vi "List Packages in SystemLink Feed.vi"(0 "SystemLink repo in":T1, 5 "feed name in":string, 11 "error in (no error)":errorcluster) -> (4 "SystemLink repo out":T1, 6 "feed name out":string, 8 "packages":string[][](table), 15 "error out":errorcluster)   [LabVIEW 2017, in "SystemLink_Repo_API.lvlib"]
doc: "Lists the packages for the specified feed.\n\nOutputs:\nPackages - This is a table (2D string array) that lists the packages in the specified feed. The table includes the name, version, filename, and package ID for each package."
uses:
  SystemLink_Repo_API.lvlib
  _support/systemlink repo.ctl
  <vilib>/httpClient/ClientHandle.ctl
  0c27402d-d134-44f2-9e9f-9c548188b8ee.vi
  73f63470-54eb-45b7-8baf-304f99d209d6.vi
  <vilib>/JDP Science/JSONtext/Find Multiple Items.vi
  <vilib>/JDP Science/JSONtext/String Subset.vi
  <vilib>/JDP Science/JSONtext/support/Strip Quotes and Unescape.vi
  <vilib>/JDP Science/JSONtext/Parsing/Parse Full Path or Item Name.vi
  <vilib>/JDP Science/JSONtext/Offset/Find Item Locations by Path.vi
  <vilib>/JDP Science/JSONtext/support/Unescape JSON string.vi
  <vilib>/JDP Science/JSONtext/JSON text to Variant.vi
  <vilib>/httpClient/LabVIEWHTTPClient.lvlib
panel:
  out "body":string
  out "headers":string
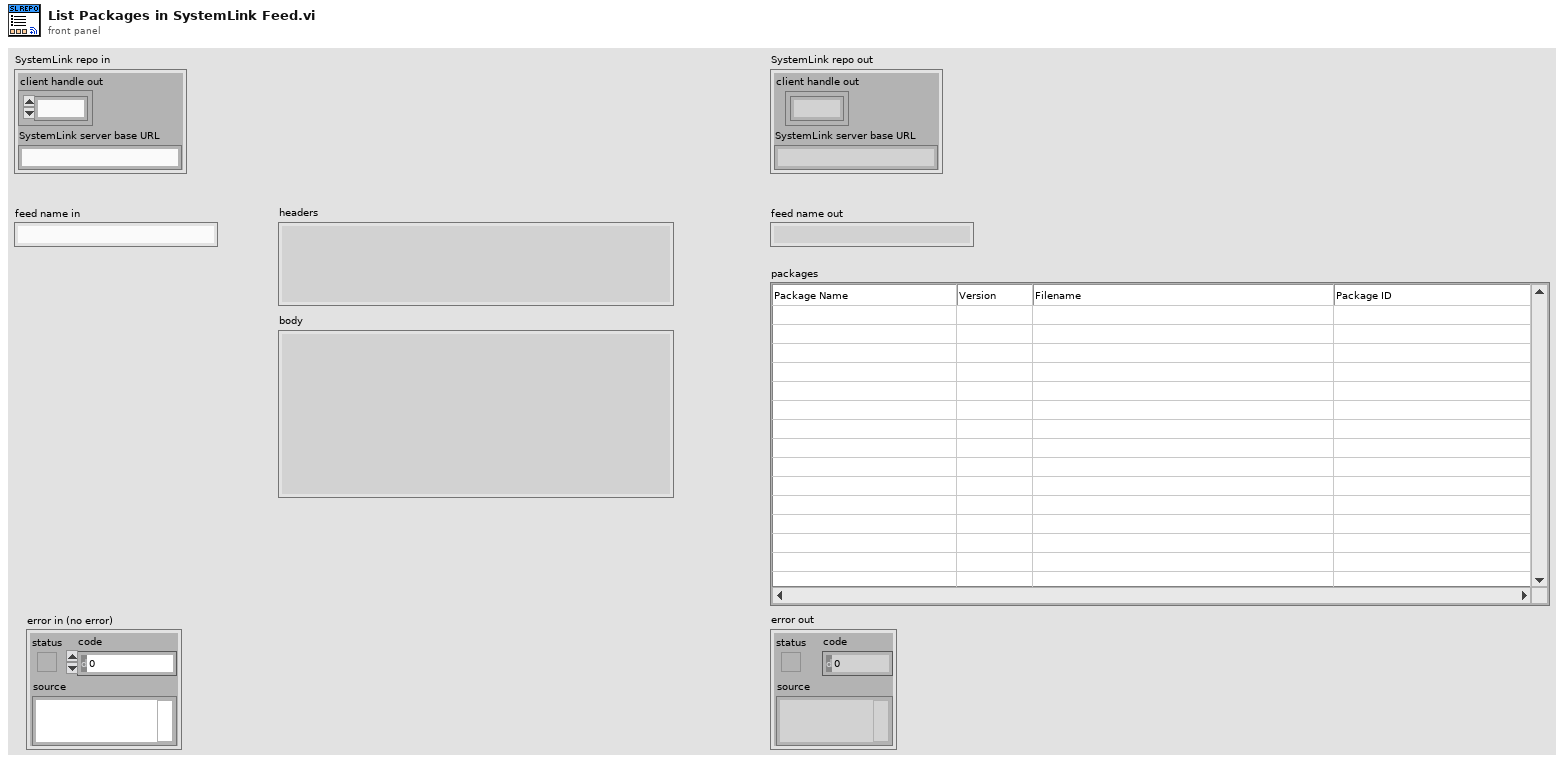
[diagram p1: front panel]
types:
  T1 = typedef "SystemLink_Repo_API.lvlib/systemlink repo.ctl" = cluster{"client handle out":T2, "SystemLink server base URL":string}
  T2 = typedef "LabVIEWHTTPClient.lvlib/ClientHandle.ctl" = refnum<k1>
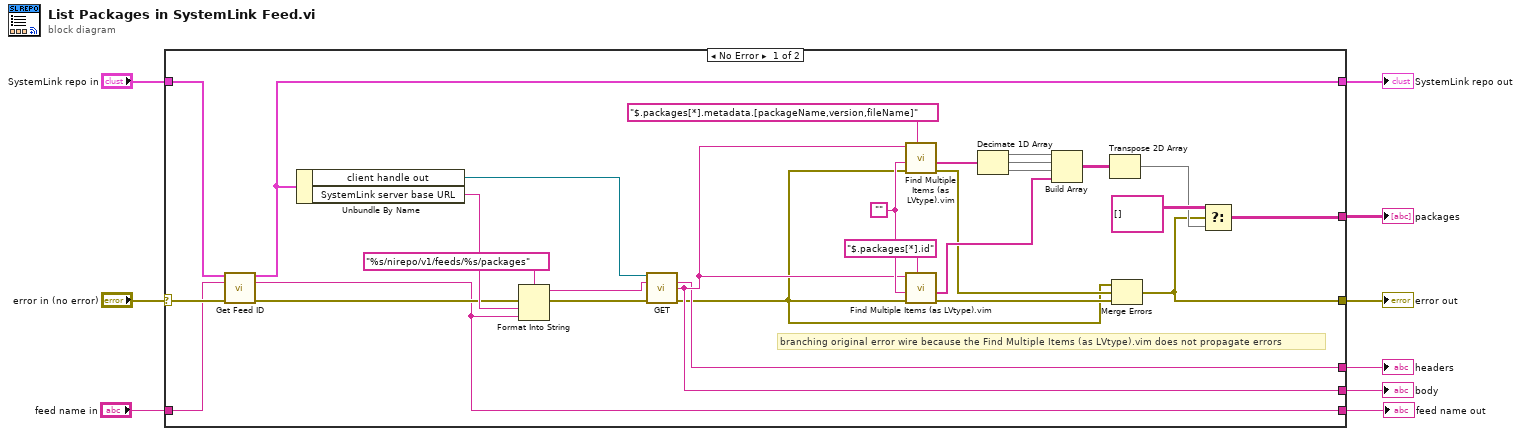
[diagram p0: block diagram]
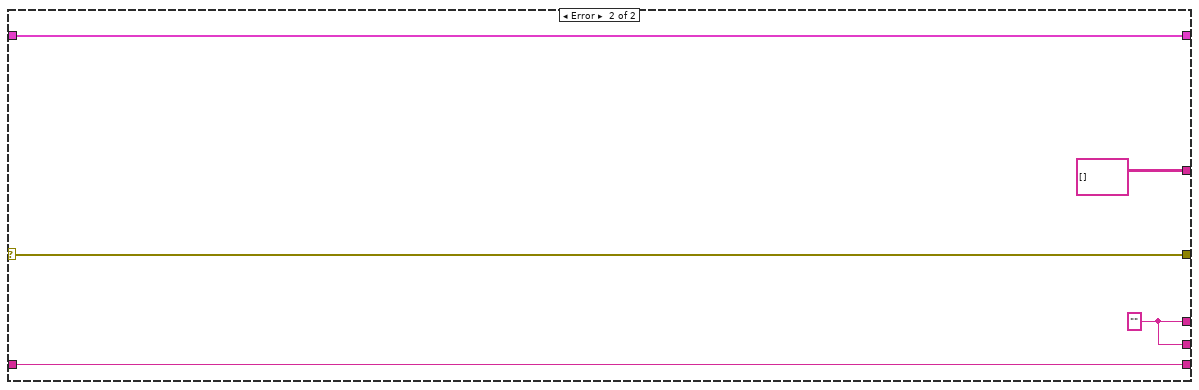
[diagram p2: hidden frame]
diagram:
  n1 = case shown="No Error" "error in (no error)" {
    selector: "error in (no error)" -> [w16 w43]
    tunnel: "SystemLink repo in" -> [w13 w40]
    tunnel: [w19 w43] -> w8
    tunnel: [w20 string[][] [] ("t")] -> w7
    tunnel: [w18 w41] -> w6
    tunnel: [w17 w41] -> w5
    tunnel: [w12 w40] -> w3
    tunnel: "feed name in" -> [w14 w39]
    tunnel: [w10 w39] -> w1
    frame No Error {
      w23 = ""
      # "branching original error wire because the Find Multiple Items (as LVtype).vim does not propagate errors"
      n2 = call "Get Feed ID.vi"("SystemLink repo in"=w13, "feed name"=w14, "error in (no error)"=w16) -> ("SystemLink repo out"=w12:T1, "feed ID"=w10:string, "error out"=w15:errorcluster)  [unwired: 10 in]
      n3 = Unbundle By Name(w12) -> ("client handle out"=w36:T2, "SystemLink server base URL"=w35:string)
      n4 = Format Into String(format string="%s/nirepo/v1/feeds/%s/packages", error in=w15, w35, w10) -> (resulting string=w37:string, error out=w34:errorcluster)  [unwired: 1 in]
      n5 = call <vilib>:"GET.vi"("client handle"=w36, "url"=w37, "error in (no error)"=w34) -> ("headers"=w17:string, "body"=w18:string, "error out"=w11:errorcluster)  [unwired: 9 in, 1 out]
      n6 = call "Find Multiple Items (as LVtype).vim"("$Path or Item Name"="$.packages[*].metadata.[packageName,version,fileName]" ("$Path for packages 2"), "error in (no error)"=w11, "Data Type and Default Value"=w23, "JSON"=w18) -> ("error out"=w25:errorcluster, "Array of Data"=w30:string[])  [unwired: 4 in, 2 out]
      n7 = call "Find Multiple Items (as LVtype).vim"("$Path or Item Name"="$.packages[*].id" ("$Path for packages"), "error in (no error)"=w11, "Data Type and Default Value"=w23, "JSON"=w18) -> ("error out"=w24:errorcluster, "Array of Data"=w26:string[])  [unwired: 4 in, 2 out]
      n8 = Decimate 1D Array(w30) -> (w29:string[], w28:string[], w27:string[])
      n9 = Build Array(w29, w28, w27, w26) -> (w31:string[][])
      n10 = Transpose 2D Array(2D array=w31) -> (transposed array=w21:string[][])
      n11 = Merge Errors(w11, w25, w24) -> (w19:errorcluster)
      n12 = Select(t=string[][] [], s=w19, f=w21) -> (s? t:f=w20:string[][])
    }
    frame Error {
      w41 = "" ("headers")
    }
  }
  "error out" <- w8
  "SystemLink repo out" <- w3
  "packages" <- w7
  "headers" <- w5
  "body" <- w6
  "feed name out" <- w1
